vi "init.vi"(8 "error in (no error)":errorcluster, 9 "RejectedCommand":refnum<user-event>, 10 "Settings.lvlib:TCSettings.lvclass":refnum<class "TCSettings.lvclass">, 11 "ElectrometerController in":refnum<class "ElectrometerController.lvclass">) -> (0 "error out":errorcluster, 3 "ElectrometerController out":refnum<class "ElectrometerController.lvclass">)   [LabVIEW 2016, in "ElectrometerController.lvclass"]
uses:
  ElectrometerController.lvclass
  ts_electrometeruserevents/ComponentTemplateCore/Settings/SettingsTC/TCSettings.lvclass
  ts_electrometeruserevents/Typedefs/RejectedCommand.ctl
  ts_electrometeruserevents/Typedefs/CommandValue.ctl
  ts_electrometeruserevents/Typedefs/StateValue.ctl
  Electrometer/internalState.ctl
  ElectrometerConfiguration/Controls/internalConfiguration.ctl
  Electrometer/AVG Filter type.ctl
  Electrometer/MED Filter Type.ctl
  Electrometer/Modes.ctl
  ElectrometerConfiguration/Controls/com_conf.ctl
  ts_electrometeruserevents/Typedefs/termChar.ctl
  Electrometer/Electrometer.lvclass
  ts_electrometeruserevents/ConfigurationTC/ConfigurationTypedefs/ConfigurationTypedefs.lvlib
  ts_electrometeruserevents/Typedefs/ElectrometerTypedefs.lvlib
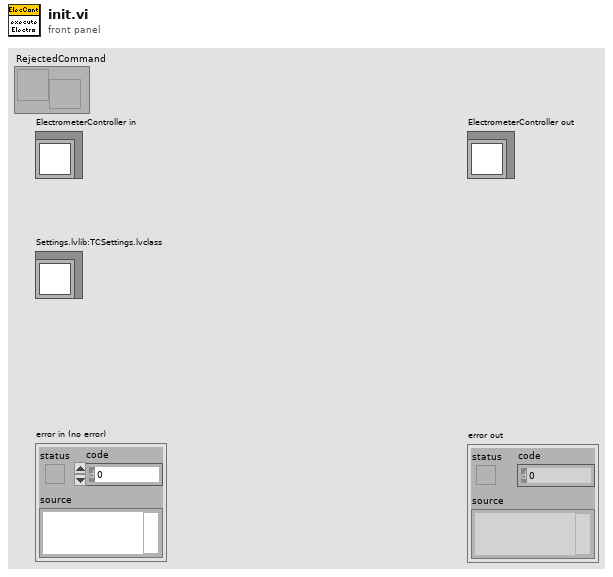
[diagram p1: front panel]
types:
  T1 = typedef "ConfigurationTypedefs.lvlib/com_conf.ctl" = cluster{"Baud Rate":dbl, "VISA resource name":refnum<visa-resource-name>, "Parity":u16, "Data Bits":u16, "Stop Bits":u16, "Flow Control":u16, "termChar":T2}
  T2 = typedef "ElectrometerTypedefs.lvlib/termChar.ctl" = enum16{"CR", "CR+LF", "LF", "LF+CR"}
  T3 = typedef "ConfigurationTypedefs.lvlib/internalConfiguration.ctl" = cluster{"IntegrationTime":dbl, " Input Range ":dbl, "Reading Option (0: Latest)":i32, "Error Path":path, "Reading Timeout":dbl, "AVG Filter type":T4, "Filter":T5, "Mode":T6, "Median Filter":T5}
  T4 = typedef "Electrometer.lvclass/AVG Filter type.ctl" = enum16{"None", "Scalar", "Advanced"}
  T5 = typedef "Electrometer.lvclass/MED Filter Type.ctl" = enum16{"Active", "None"}
  T6 = typedef "Electrometer.lvclass/Modes.ctl" = enum16{"Current", "Charge"}
  T7 = typedef "Electrometer.lvclass/internalState.ctl" = enum16{"Ready", "Configuring", "ManualReading", "UntilIntensityReading", "SetDurationReading"}
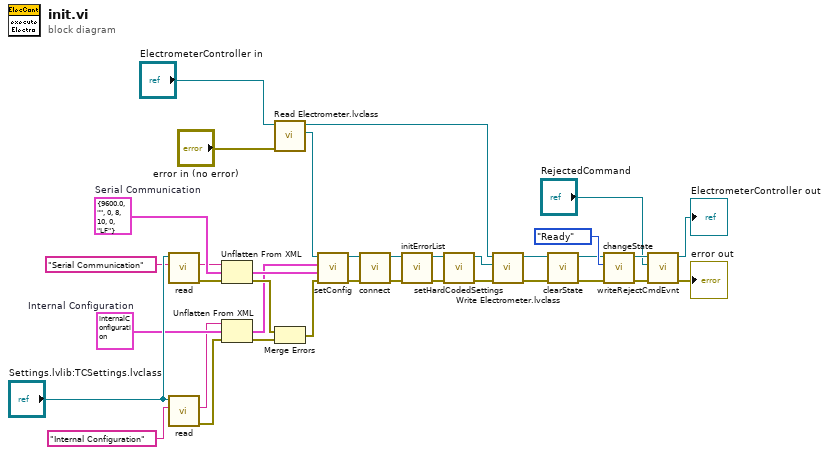
[diagram p0: block diagram]
diagram:
  w15 = T1 {"Baud Rate"=9600.0, "VISA resource name"="", "Parity"=0, "Data Bits"=8, "Stop Bits"=10, "Flow Control"=0, "termChar"=enum."LF"}  # Serial Communication
  w19 = T3 {"IntegrationTime"=0.002, " Input Range "=10.0, "Reading Option (0: Latest)"=0, "Error Path"=path "", "Reading Timeout"=600.0, "AVG Filter type"=enum."None", "Filter"=enum."None", "Mode"=enum."Current", "Median Filter"=enum."Active"}  # Internal Configuration
  n1 = call-dynamic "read.vi"("Name"="Serial Communication", "BaseSetting in"="Settings.lvlib:TCSettings.lvclass") -> ("error out"=w13:errorcluster, "XML"=w14:string)  [unwired: 6 in, 2 out]
  n2 = call-dynamic "read.vi"("Name"="Internal Configuration", "BaseSetting in"="Settings.lvlib:TCSettings.lvclass") -> ("error out"=w17:errorcluster, "XML"=w18:string)  [unwired: 6 in, 2 out]
  n3 = Unflatten From XML(xml string=w14, type=w15, error in (no error)=w13) -> (value=w11:T1, error out=w12:errorcluster)
  n4 = Unflatten From XML(xml string=w18, type=w19, error in (no error)=w17) -> (value=w10:T3, error out=w16:errorcluster)
  n5 = call-dynamic "Read Electrometer.lvclass.vi"("error in (no error)"="error in (no error)", "ElectrometerController in"="ElectrometerController in") -> ("Electrometer.lvclass"=w31:refnum<class "Electrometer.lvclass">, "ElectrometerController out"=w29:refnum<class "ElectrometerController.lvclass">)  [unwired: 7 in, 1 out]
  n6 = Merge Errors(w12, w16) -> (w20:errorcluster)
  n7 = call-dynamic "setConfig.vi"("error in (no error)"=w20, "Serial Communication"=w11, "Internal Configuration"=w10, "Electrometer in"=w31) -> ("error out"=w24:errorcluster, "Electrometer out"=w36:refnum<class "Electrometer.lvclass">)  [unwired: 6 in]
  n8 = call "connect.vi"("error in (no error)"=w24, "Electrometer in"=w36) -> ("error out"=w35:errorcluster, "Electrometer out"=w34:refnum<class "Electrometer.lvclass">)  [unwired: 7 in, 1 out]
  n9 = call-dynamic "initErrorList.vi"("error in (no error)"=w35, "Electrometer in"=w34) -> ("error out"=w3:errorcluster, "Electrometer out"=w4:refnum<class "Electrometer.lvclass">)  [unwired: 8 in]
  n10 = call "setHardCodedSettings.vi"("error in (no error)"=w3, "Electrometer in"=w4) -> ("error out"=w2:errorcluster, "Electrometer out"=w1:refnum<class "Electrometer.lvclass">)  [unwired: 8 in]
  n11 = call-dynamic "Write Electrometer.lvclass.vi"("error in (no error)"=w2, "Electrometer.lvclass"=w1, "ElectrometerController in"=w29) -> ("error out"=w25:errorcluster, "ElectrometerController out"=w28:refnum<class "ElectrometerController.lvclass">)  [unwired: 7 in]
  n12 = call "clearState.vi"("error in (no error)"=w25, "ElectrometerController in"=w28) -> ("error out"=w26:errorcluster, "ElectrometerController out"=w27:refnum<class "ElectrometerController.lvclass">)  [unwired: 8 in]
  n13 = call "changeState.vi"("error in (no error)"=w26, "State"=internalState."Ready" ("States"), "ElectrometerController in"=w27) -> ("error out"=w8:errorcluster, "ElectrometerController out"=w9:refnum<class "ElectrometerController.lvclass">)  [unwired: 7 in]
  n14 = call "writeRejectCmdEvnt.vi"("error in (no error)"=w8, "RejectedCommand"="RejectedCommand", "ElectrometerController in"=w9) -> ("error out"=→"error out":errorcluster, "ElectrometerController out"=→"ElectrometerController out":refnum<class "ElectrometerController.lvclass">)  [unwired: 7 in]
